vi "NI VeriStand - Write Single Waveform (CDB).vi"(8 "error in (no error)":errorcluster, 9 "timeout in ms (0)":i32, 10 "Data":cdb[](array[numeric]), 11 "Single Waveform Write Session (CDB) in":refnum<class "Single Waveform Write (CDB).lvclass">) -> (0 "error out":errorcluster, 1 "timed out?":bool, 3 "Single Waveform Write Session (CDB) out":refnum<class "Single Waveform Write (CDB).lvclass">)   [LabVIEW 2020, in "NI_VS Custom Device Waveform API.lvlib" / "Single Waveform Write (CDB).lvclass"]
doc: "Writes an array of values to the waveform(s) associated with the specified write session. Use the Start Waveform(s) VI prior to this VI to set the waveform start time (t0) or start times. NI VeriStand considers all data this VI writes to be continuous unless the Start Waveform(s) VI executes again with a different start time."
uses:
  Single Waveform Write (CDB).lvclass
  D:/p4/penguin/lvaddon/Veristand/master/src/LabVIEW/vilib/NI VeriStand/Custom Device Waveform API/Waveform Session.lvclass
  Waveform Session.lvclass/Waveform Session.ctl
  Single Waveform Write (CDB).lvclass/Single Waveform Write (CDB).ctl
  Internal Comm Classes/WPL Comm/WPL Comm (1D CDB)/WPL Comm (1D CDB).lvclass/WPL Comm (1D CDB).ctl
  Internal Comm Classes/WPL Comm/WPL Comm.lvclass/WPL Comm.ctl
  Internal Comm Classes/WPL Comm/Direct Send WPL Command.vi
  Internal Comm Classes/WPL Comm/Convert Q Error to Shutdown Error.vi
  Internal Comm Classes/WPL Comm/WPL Comm (1D CDB)/WPL Comm (1D CDB).lvclass
  D:/p4/penguin/lvaddon/Veristand/master/src/LabVIEW/vilib/NI VeriStand/Custom Device Waveform API/Internal Comm Classes/WPL Comm/WPL Comm.lvclass
  <vilib>/Utility/error.llb/Error Cluster From Error Code.vi
  Waveform Session.lvclass
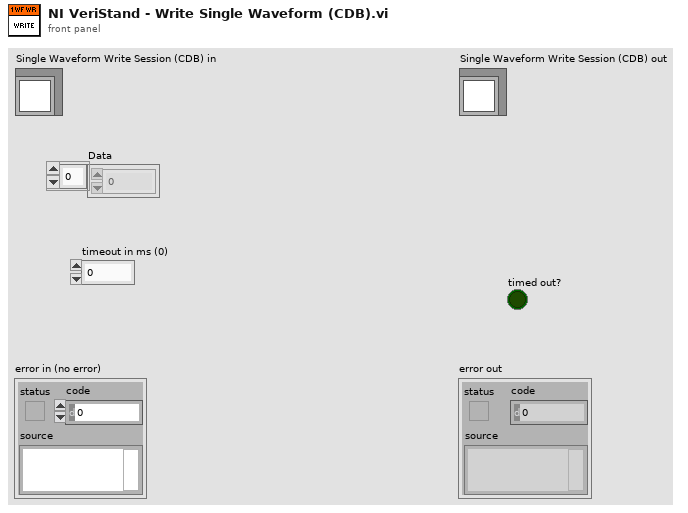
[diagram p1: front panel]
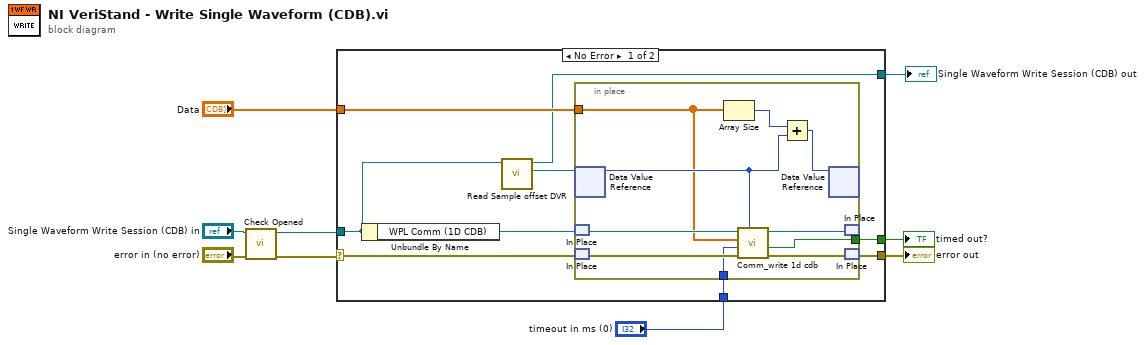
[diagram p0: block diagram]
diagram:
  n1 = call "Check Opened.vi"("error in (no error)"="error in (no error)", "Waveform Session in"="Single Waveform Write Session (CDB) in") -> ("error out"=w2:errorcluster, "Waveform Session out"=w1:refnum<class "Single Waveform Write (CDB).lvclass">)  [unwired: 8 in]
  n2 = case shown="No Error" w2 {
    selector: w2 -> [w12 w30]
    tunnel: [w18 w30] -> w9
    tunnel: [w13 w29] -> w8
    tunnel: "Data" -> [w17 _]
    tunnel: [w16 _] -> w7
    tunnel: "timeout in ms (0)" -> [w15 _]
    tunnel: w1 -> [w11 w29]
    frame No Error {
      n3 = Unbundle By Name(w11) -> ("WPL Comm (1D CDB)"=w10:refnum<class "WPL Comm (1D CDB).lvclass">)
      n4 = call "Read Sample offset DVR.vi"("Waveform Session in"=w11) -> ("Sample offset"=w14:refnum<data-value>, "Waveform Session out"=w13:refnum<class "Single Waveform Write (CDB).lvclass">)  [unwired: 9 in]
      n5 = in-place {
        in-place-border: w17 -> [w20]
        in-place-border: [w23] -> w16
        in-place-border: w15 -> [w22]
        n6 = in-place-dvr #1(w14) -> (w21:u64)  [unwired: 1 out]
        n7 = in-place-match #2(w10) -> (w26:refnum<class "WPL Comm (1D CDB).lvclass">)
        n8 = in-place-match #3(w12) -> (w27:errorcluster)
        n9 = Array Size(array=w20) -> (size(s)=w19:i32)
        n10 = call "Comm_write 1d cdb.vi"("Sample Offset"=w21, "error in (no error)"=w27, "timeout in ms (0)"=w22, "Data"=w20, "WPL Comm (1D CDB) in"=w26) -> ("error out"=w24:errorcluster, "timed out?"=w23:bool, "WPL Comm (1D CDB) out"=w25:refnum<class "WPL Comm (1D CDB).lvclass">)  [unwired: 4 in]
        n11 = Add(x=w19, y=w21) -> (x+y=w28:u64)
        n12 = in-place-dvr #1(w28) -> ()  [unwired: 2 out]
        n13 = in-place-match #2(w25) -> ()  [unwired: 1 out]
        n14 = in-place-match #3(w24) -> (w18:errorcluster)
      }
    }
    frame Error {
    }
  }
  "error out" <- w9
  "Single Waveform Write Session (CDB) out" <- w8
  "timed out?" <- w7
